vi "ImageDataFlush.vi"(8 "error in (no error)":errorcluster, 11 "Image in":refnum<class "Image.lvclass">) -> (0 "error out":errorcluster, 3 "Image out":refnum<class "Image.lvclass">)   [LabVIEW 2012, in "Image.lvclass"]
uses:
  classes/Image.lvclass
  classes/Image.lvclass/Image.ctl
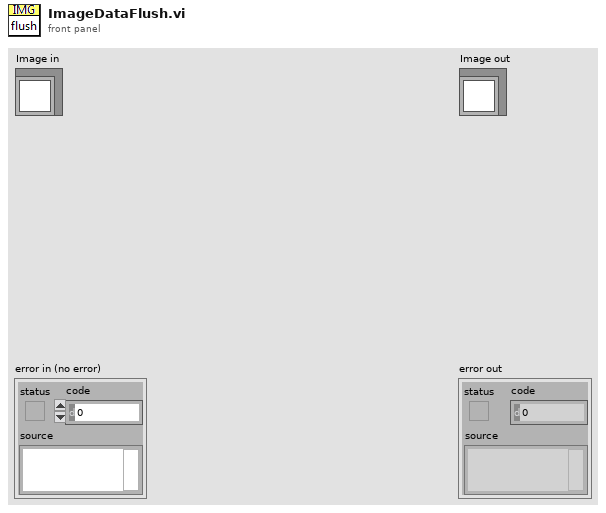
[diagram p1: front panel]
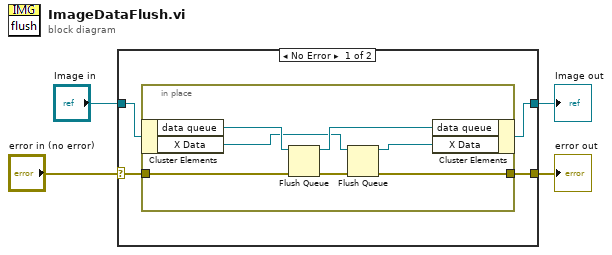
[diagram p0: block diagram]
diagram:
  n1 = case shown="No Error" "error in (no error)" {
    selector: "error in (no error)" -> [w6 w17]
    tunnel: [w5 w17] -> w3
    tunnel: [w7 w16] -> w1
    tunnel: "Image in" -> [w8 w16]
    frame No Error {
      n2 = in-place {
        in-place-border: w6 -> [w11]
        in-place-border: [w9] -> w5
        n3 = in-place-cluster #1(w8) -> ("data queue"=w15:refnum<queue>, "X Data"=w13:refnum<queue>)
        n4 = Flush Queue(queue=w15, error in (no error)=w11) -> (queue out=w14:refnum<queue>, error out=w10:errorcluster)  [unwired: 1 out]
        n5 = Flush Queue(queue=w13, error in (no error)=w10) -> (queue out=w12:refnum<queue>, error out=w9:errorcluster)  [unwired: 1 out]
        n6 = in-place-cluster #1("data queue"=w14, "X Data"=w12) -> (w7:refnum<class "Image.lvclass">)
      }
    }
    frame Error {
    }
  }
  "error out" <- w3
  "Image out" <- w1
